vi "Log Result.vi"(8 "error in (no error)":errorcluster, 10 "Result":refnum<class "Acquired Result.lvclass">, 11 "Logger in":refnum<class "Logger.lvclass">) -> (0 "error out":errorcluster, 3 "Logger out":refnum<class "Logger.lvclass">)   [LabVIEW 2016, in "Logger.lvclass"]
uses:
  Logger.lvclass
  NHMFL_Core/Libraries/Instruments/Results/Acquired Result/Acquired Result.lvclass
  Logger.lvclass/Logger.ctl
  Read File.lvclass.vi
  Read Last clean-up time stamp.vi
  Read Clean-up period.vi
  Write File.lvclass.vi
  Write Last clean-up time stamp.vi
  NHMFL_Core/Libraries/File/File Class/File.lvclass
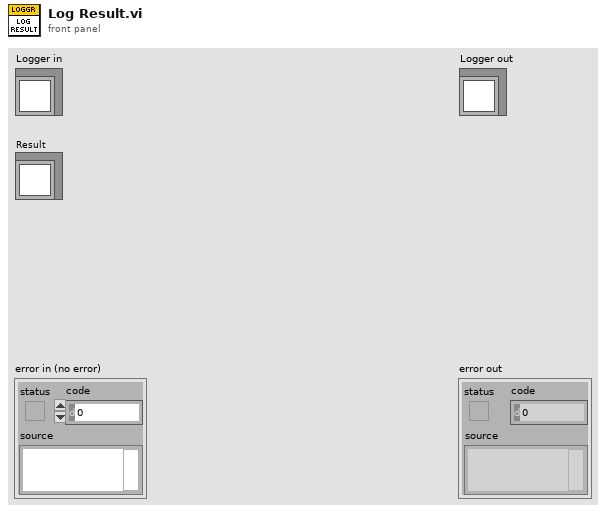
[diagram p1: front panel]
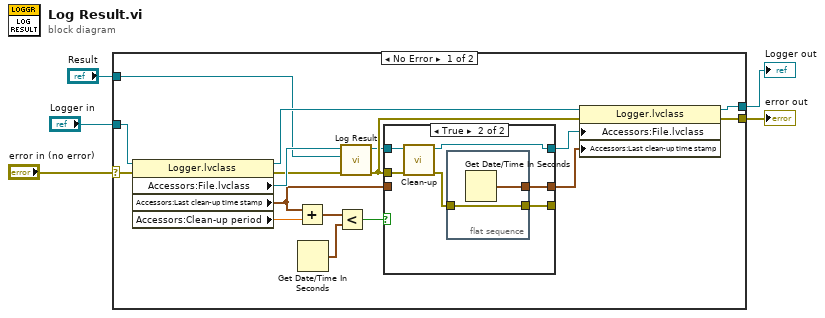
[diagram p0: block diagram]
diagram:
  n1 = case shown="No Error" "error in (no error)" {
    selector: "error in (no error)" -> [w22 w35]
    tunnel: [w20 w35] -> w4
    tunnel: [w18 w34] -> w2
    tunnel: "Logger in" -> [w21 w34]
    tunnel: "Result" -> [w15 _]
    frame No Error {
      n2 = property class="Logger.lvclass"(reference=w21, error in=w22) -> (reference out=w19:refnum<class "Logger.lvclass">, error out=w16:errorcluster, "Accessors:File.lvclass"=w17:refnum<class "File.lvclass">, "Accessors:Last clean-up time stamp"=w7:timestamp, "Accessors:Clean-up period"=w14:dbl)
      n3 = Add(x=w7, y=w14) -> (x+y=w12:timestamp)
      n4 = Get Date/Time In Seconds() -> (seconds since 1Jan1904=w13:timestamp)
      n5 = Less?(x=w12, y=w13) -> (x < y?=w11:bool)
      n6 = call-dynamic "Log Result.vi"("error in (no error)"=w16, "Result"=w15, "File in"=w17) -> ("error out"=w10:errorcluster, "File out"=w9:refnum<class "File.lvclass">)  [unwired: 7 in]
      n7 = case shown="True" w11 {
        tunnel: w10 -> [w25 w31]
        tunnel: w9 -> [w24 w30]
        tunnel: [w25 w26] -> _
        tunnel: [w24 w29] -> w8
        tunnel: w7 -> [w23 _]
        tunnel: [w23 w28] -> w6
        frame False {
        }
        frame True {
          n8 = call-dynamic "Clean-up.vi"("error in (no error)"=w31, "File in"=w30) -> ("error out"=w27:errorcluster, "File out"=w29:refnum<class "File.lvclass">)  [unwired: 8 in]
          n9 = flat-sequence {
            tunnel: [w33] -> w28
            tunnel: w27 -> [w32]
            tunnel: [w32] -> w26
            frame #0 {
              n10 = Get Date/Time In Seconds() -> (seconds since 1Jan1904=w33:timestamp)
            }
          }
        }
      }
      n11 = property class="Logger.lvclass"(reference=w19, error in=w10, "Accessors:File.lvclass"=w8, "Accessors:Last clean-up time stamp"=w6) -> (reference out=w18:refnum<class "Logger.lvclass">, error out=w20:errorcluster)
    }
    frame Error {
    }
  }
  "error out" <- w4
  "Logger out" <- w2
